vi "ep_Check Speed Value.vi"(8 "error in (no error)":errorcluster, 11 "speed [RPM]":dbl) -> (0 "error out":errorcluster)   [LabVIEW 2014, in "NI_EP_Motor Monitoring.lvlib"]
uses:
  <vilib>/addons/Electrical Power/Motor Monitoring/NI_EP_Motor Monitoring.lvlib
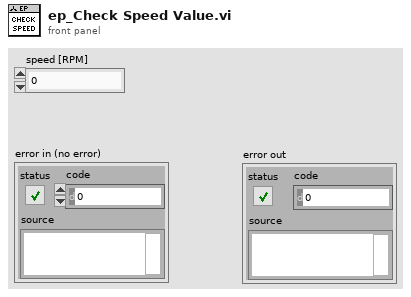
[diagram p1: front panel]
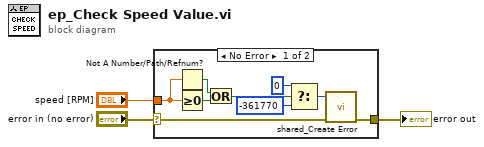
[diagram p0: block diagram]
diagram:
  n1 = case shown="No Error" "error in (no error)" {
    selector: "error in (no error)" -> [w9 w13]
    tunnel: [w8 w13] -> w2
    tunnel: "speed [RPM]" -> [w5 _]
    frame No Error {
      n2 = Not A Number/Path/Refnum?(number/path/refnum=w5) -> (NaN/Path/Refnum?=w4:bool)
      n3 = Greater Or Equal To 0?(x=w5) -> (x >= 0?=w6:bool)
      n4 = Or(x=w4, y=w6) -> (x .or. y?=w12:bool)
      n5 = Select(t=0, s=w12, f=-361770 ("error code (0)")) -> (s? t:f=w7:i32)
      n6 = call <vilib>:"shared_Create Error.vi"("error in (no error)"=w9, "error code (0)"=w7) -> ("error out"=w8:errorcluster)  [unwired: 9 in]
    }
    frame Error {
    }
  }
  "error out" <- w2
